vi "Create.vi"(8 "Error In":errorcluster, 10 "Tag":string, 11 "Pixel In":refnum<class "Pixel.lvclass">) -> (0 "Error Out":errorcluster, 3 "Pixel":refnum<class "Pixel.lvclass">)   [LabVIEW 2019, in "Pixel.lvclass"]
uses:
  Pixel.lvclass
  Display Element/Display Element.lvclass
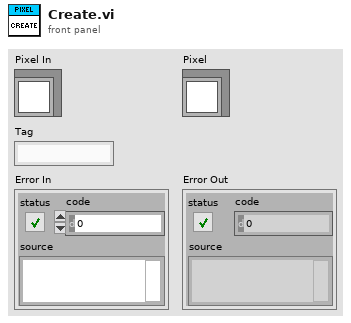
[diagram p1: front panel]
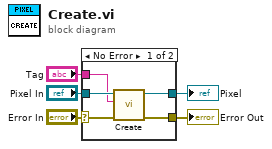
[diagram p0: block diagram]
diagram:
  n1 = case shown="No Error" "Error In" {
    selector: "Error In" -> [w8 w11]
    tunnel: [w10 w11] -> w5
    tunnel: [w9 w12] -> w4
    tunnel: "Pixel In" -> [w7 w12]
    tunnel: "Tag" -> [w6 _]
    frame No Error {
      n2 = call-parent "Create.vi"("Error In"=w8, "Tag"=w6, "Display Element In"=w7) -> ("Error Out"=w10:errorcluster, "Display Element"=w9:refnum<class "Pixel.lvclass">)  [unwired: 7 in]
    }
    frame Error {
    }
  }
  "Pixel" <- w4
  "Error Out" <- w5
